vi "Write Parameter to Word.vi"(8 "error in":errorcluster, 9 "parameter definition":T1={"start index"=10, "size"=19, "encoding"=enum."BNR", "signed"=FALSE, "scale multiplier"=1.0, "scale offset"=0.0}, 10 "data":dbl, 11 "32-bit Word in":refnum<class "32-bit Word.lvclass">) -> (0 "error out":errorcluster, 3 "32-bit Word out":refnum<class "32-bit Word.lvclass">)   [LabVIEW 2020, in "32-bit Word.lvclass"]
uses:
  32-bit Word.lvclass
  Parameter Definition.ctl
  Encoding and Decoding/Encoding.ctl
  32-bit Word.lvclass/32-bit Word.ctl
  a9fc36c8-445f-4369-8da7-39f8ca0e4fb3.vi
  18ae2359-2592-47e8-a0f7-10a9dc742aaf.vi
  Read 32-Bit Word.vi
  Write 32-Bit Word.vi
  a9fc36c8-445f-4369-8da7-39f8ca0e4fb3.vi/9377bb8f-44b5-4a8f-87f1-966fd5a9edcc.vi
  18ae2359-2592-47e8-a0f7-10a9dc742aaf.vi/a54b505c-1216-4ef4-8378-3ceda9d188df.vi
  18ae2359-2592-47e8-a0f7-10a9dc742aaf.vi/136dcdcb-2dd3-4a4d-a796-a8f7a3f8e1ac.vi
  18ae2359-2592-47e8-a0f7-10a9dc742aaf.vi/a54b505c-1216-4ef4-8378-3ceda9d188df.vi/a7fcce85-1f75-4572-aeaa-ddfd463a7c5f.vi
  ARINC 429.lvclass
  Encoding and Decoding/Encoding and Decoding.lvlib
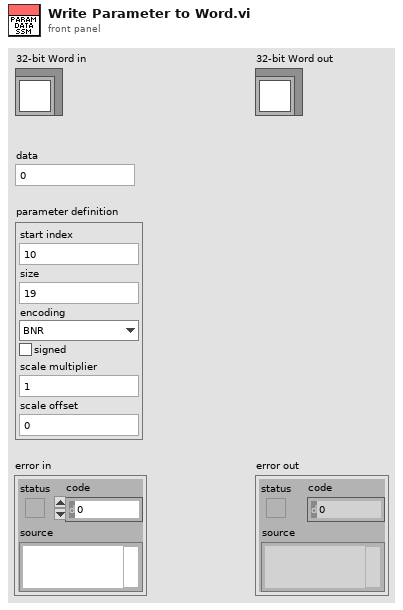
[diagram p1: front panel]
types:
  T1 = typedef "ARINC 429.lvclass/Parameter Definition.ctl" = cluster{"start index":i32, "size":i32, "encoding":T2, "signed":bool, "scale multiplier":dbl, "scale offset":dbl}
  T2 = typedef "Encoding and Decoding.lvlib/Encoding.ctl" = enum16{"BNR", "BCD", "Discrete"}
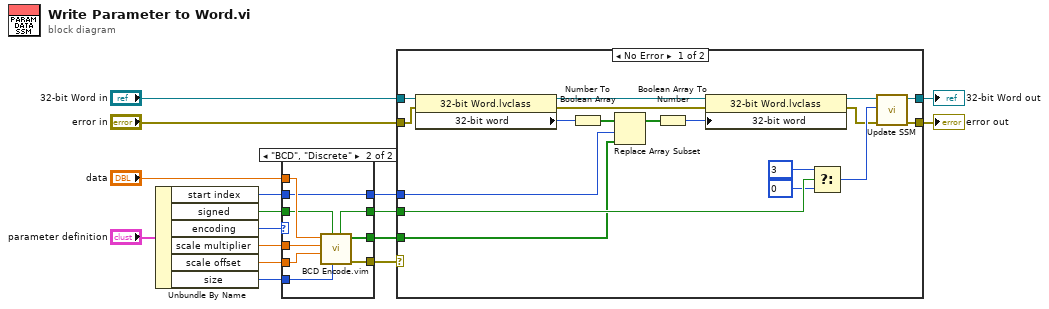
[diagram p0: block diagram]
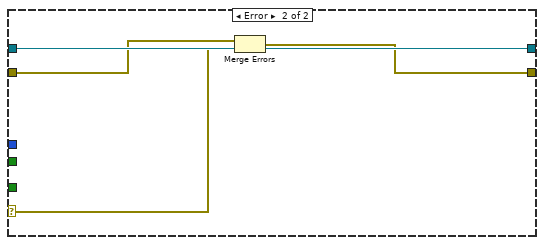
[diagram p2: hidden frame]
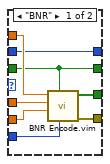
[diagram p3: hidden frame]
diagram:
  n1 = Unbundle By Name("parameter definition") -> ("start index"=w1:i32, "signed"=w8:bool, "encoding"=w13:T2, "scale multiplier"=w11:dbl, "scale offset"=w10:dbl, "size"=w9:i32)
  n2 = case shown="\"BCD\", \"Discrete\"" w13 {
    tunnel: "data" -> [w24 w33]
    tunnel: w11 -> [w23 w32]
    tunnel: w10 -> [w22 w31]
    tunnel: w9 -> [w21 w28]
    tunnel: w8 -> [w18 w30]
    tunnel: [w18 w29] -> w7
    tunnel: [w20 w27] -> w6
    tunnel: [w19 w26] -> w3
    tunnel: [w17 w25] -> w2
    tunnel: w1 -> [w17 w25]
    frame "BNR" {
      n3 = call "BNR Encode.vim"("data size (bits)"=w21, "signed"=w18, "scale offset"=w22, "scale multiplier"=w23, "value"=w24) -> ("error out"=w19:errorcluster, "BNR encoded value"=w20:bool[])  [unwired: 5 in]
    }
    frame "BCD", "Discrete" {
      n4 = call "BCD Encode.vim"("data size (bits)"=w28, "signed"=w30, "scale offset"=w31, "scale multiplier"=w32, "value"=w33) -> ("error out"=w26:errorcluster, "BCD encoded value"=w27:bool[], "signed?"=w29:bool)  [unwired: 4 in]
    }
  }
  n5 = case shown="No Error" w3 {
    selector: w3 -> [_ w53]
    tunnel: "32-bit Word in" -> [w51 w55]
    tunnel: [w50 w55] -> w15
    tunnel: w7 -> [w48 _]
    tunnel: w2 -> [w43 _]
    tunnel: w6 -> [w42 _]
    tunnel: "error in" -> [w36 w54]
    tunnel: [w34 w52] -> w4
    frame No Error {
      n6 = property on="Property Node" class="32-bit Word.lvclass"(reference=w51, error in=w36) -> (reference out=w40:refnum<class "32-bit Word.lvclass">, error out=w37:errorcluster, "32-bit word"=w49:u32)
      n7 = Number To Boolean Array(number=w49) -> (Boolean array=w44:bool[])
      n8 = Replace Array Subset(array=w44, new element=w42, index=w43) -> (w41:bool[])
      n9 = Boolean Array To Number(Boolean array=w41) -> (number=w38:u32)
      n10 = property on="Property Node" class="32-bit Word.lvclass"(reference=w40, error in=w37, "32-bit word"=w38) -> (reference out=w39:refnum<class "32-bit Word.lvclass">, error out=w35:errorcluster)
      n11 = Select(t=u8 3 ("SDI value"), s=w48, f=u8 0 ("SDI value")) -> (s? t:f=w45:u8)
      n12 = call-dynamic "Update SSM.vi"("error in"=w35, "SSM value"=w45, "32-bit Word in"=w39) -> ("error out"=w34:errorcluster, "32-bit Word out"=w50:refnum<class "32-bit Word.lvclass">)  [unwired: 7 in]
    }
    frame Error {
      n13 = Merge Errors(w54, w53) -> (w52:errorcluster)
    }
  }
  "error out" <- w4
  "32-bit Word out" <- w15
